vi "Untitled 11.vi"(8 "error in (no error)":errorcluster, 9 "MSG":string, 10 "MSG Status":bool, 11 "Domino Laser module Class in":refnum<class "Domino Laser module Class.lvclass">) -> (0 "error out":errorcluster, 3 "Domino Laser module Class out":refnum<class "Domino Laser module Class.lvclass">)   [LabVIEW 2015, in "Domino LM.lvlib" / "Domino Laser module Class.lvclass"]
uses:
  Domino Laser module Class.lvclass
  Domino Laser module Class.lvclass/Domino Laser module Class.ctl
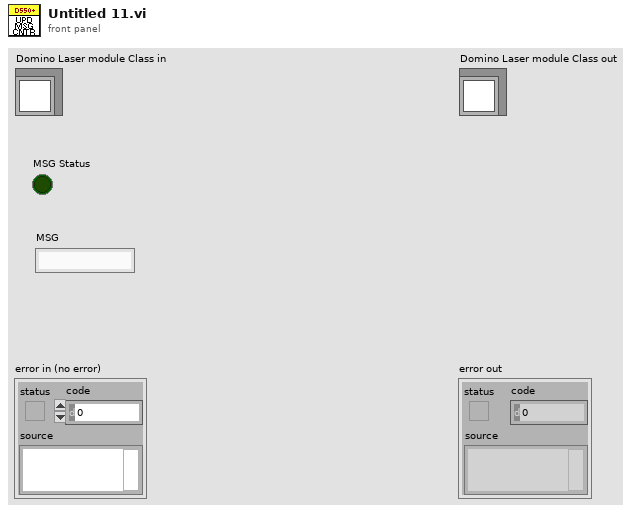
[diagram p1: front panel]
types:
  T1 = cluster{"Error Led":bool[], "Error MSG":string[]}
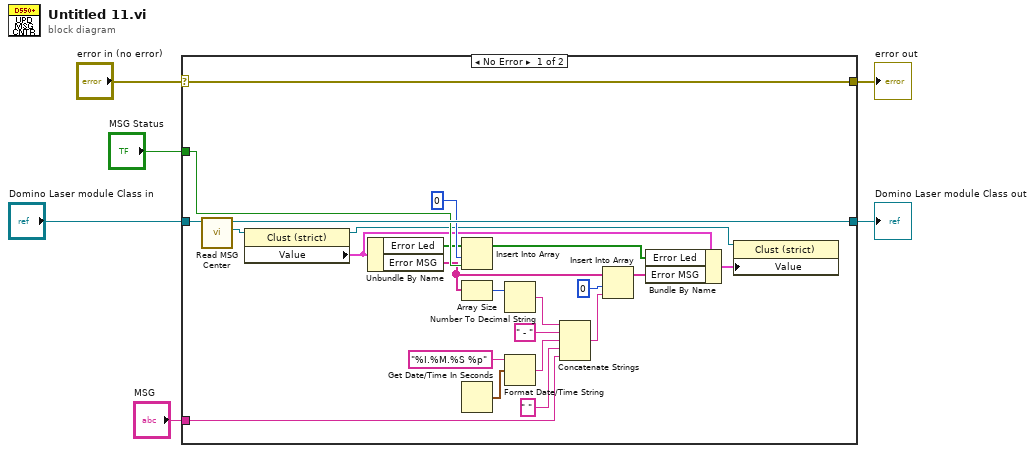
[diagram p0: block diagram]
diagram:
  n1 = case shown="No Error" "error in (no error)" {
    selector: "error in (no error)" -> [w29 w31]
    tunnel: [w29 w31] -> w5
    tunnel: [w27 w30] -> w3
    tunnel: "Domino Laser module Class in" -> [w28 w30]
    tunnel: "MSG Status" -> [w24 _]
    tunnel: "MSG" -> [w8 _]
    frame No Error {
      n2 = call "Read MSG Center.vi"("Domino Laser module Class in"=w28) -> ("MSG Center"=w26:refnum<vi>, "Domino Laser module Class out"=w27:refnum<class "Domino Laser module Class.lvclass">)  [unwired: 8 in, 1 out]
      n3 = property class="Clust (strict)"(reference=w26) -> (reference out=w13:refnum<vi>, "Value"=w17:T1)  [unwired: 1 in, 1 out]
      n4 = Unbundle By Name(w17) -> ("Error Led"=w23:bool[], "Error MSG"=w21:string[])
      n5 = Insert Into Array(array=w23, index=0, new element=w24) -> (w16:bool[])
      n6 = Array Size(array=w21) -> (size(s)=w20:i32)
      n7 = Get Date/Time In Seconds() -> (seconds since 1Jan1904=w11:timestamp)
      n8 = Number To Decimal String(number=w20) -> (decimal integer string=w19:string)  [unwired: 1 in]
      n9 = Format Date/Time String(time format string (%c)="%I.%M.%S %p", seconds (now)=w11) -> (date/time string=w10:string)  [unwired: 1 in]
      n10 = Concatenate Strings(w19, " - " ("string"), w10, " " ("string"), w8) -> (w7:string)
      n11 = Insert Into Array(array=w21, index=0, new element=w7) -> (w15:string[])
      n12 = Bundle By Name(cluster=w17, "Error Led"=w16, "Error MSG"=w15) -> (w14:T1)
      n13 = property class="Clust (strict)"(reference=w13, "Value"=w14) -> ()  [unwired: 1 in, 2 out]
    }
    frame Error {
    }
  }
  "error out" <- w5
  "Domino Laser module Class out" <- w3
